vi "Sr530 ChaînePar.vi"(8 "entrée d'erreur (pas d'erreur)":errorcluster, 11 "LockInPar":T1={"BandFilter"=FALSE, "LineFilter1x"=FALSE, "LineFilter2x"=FALSE, "Expand Ch1"=FALSE, "Expand Ch2"=FALSE, "Sensitivity"=1, "Pre Time"=1, "Post Time"=0, "Dynamic Res."=0, "Reference Trigger"=0, "Channels Settings"=0, "Frequency"=0.0} caption="Lock-In Parameters" {"Channels Settings" items=["X, Y", "X Offset, Y Offset", "R, Teta", "R Offset, Teta", "X Noise, Y Noise", "X5 (D/A), X6 (D/A)"]; "Reference Trigger" items=["Positive", "Symmetric", "Negative"]; "Post Time" items=["None", "0.1 s", "1 s"]; "Pre Time" items=["1 ms"=1, "3 ms"=2, "10 ms"=3, "30 ms"=4, "100 ms"=5, "300 ms"=6, "1 s"=7, "3 s"=8, "10 s"=9, "30 s"=10, "100 s"=11]; "Sensitivity" items=["10 nV"=1, "20 nV"=2, "50 nV"=3, "100 nV"=4, "200 nV"=5, "500 nV"=6, "1 µV"=7, "2 µV"=8, "5 µV"=9, "10 µV"=10, "20 µV"=11, "50 µV"=12, "100µV"=13, "200 µV"=14, "500µV"=15, "1 mV"=16, "2 mV"=17, "5 mV"=18, "10 mV"=19, "20 mV"=20, "50 mV"=21, "100 mV"=22]; "Dynamic Res." items=["Low", "Normal", "High"]}) -> (0 "sortie d'erreur":errorcluster, 3 "Chaîne":string)   [LabVIEW 2019]
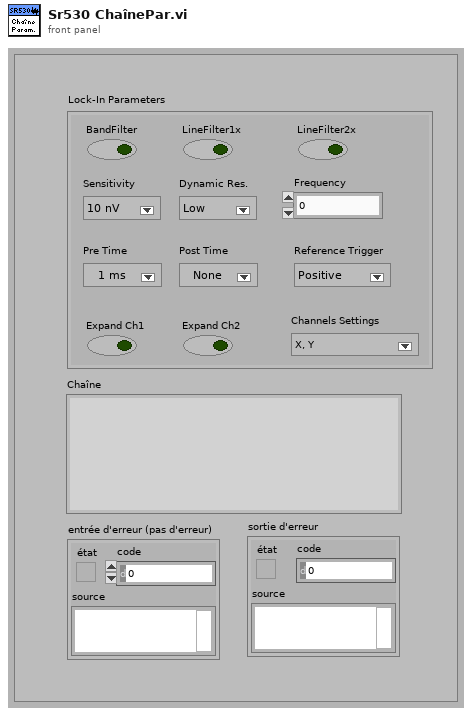
[diagram p1: front panel]
types:
  T1 = cluster{"BandFilter":bool, "LineFilter1x":bool, "LineFilter2x":bool, "Expand Ch1":bool, "Expand Ch2":bool, "Sensitivity":u16, "Pre Time":u16, "Post Time":u16, "Dynamic Res.":u16, "Reference Trigger":u16, "Channels Settings":u16, "Frequency":dbl}
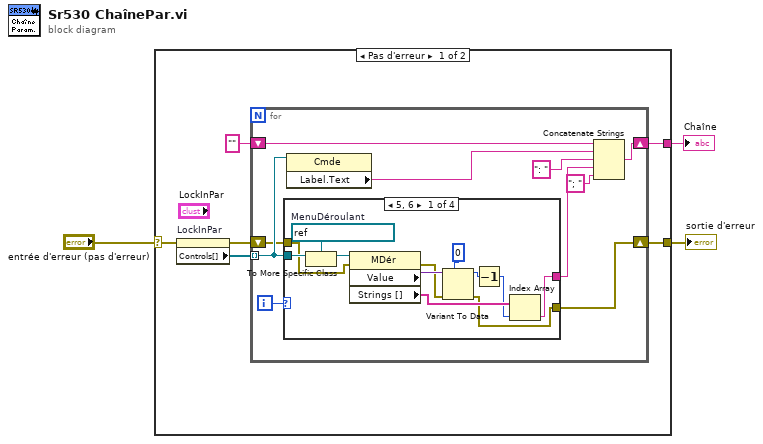
[diagram p0: block diagram]
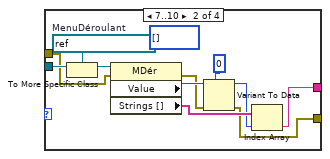
[diagram p2: hidden frame]
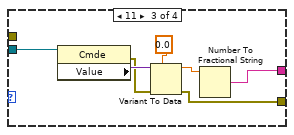
[diagram p3: hidden frame]
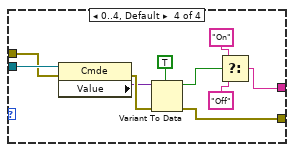
[diagram p4: hidden frame]
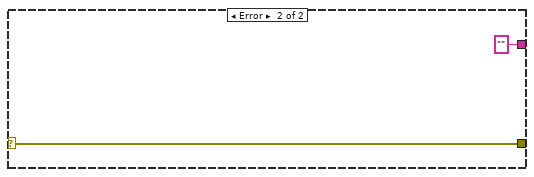
[diagram p5: hidden frame]
diagram:
  n1 = case shown="Pas d'erreur" "entrée d'erreur (pas d'erreur)" {
    selector: "entrée d'erreur (pas d'erreur)" -> [w4 w61]
    tunnel: [w7 ""] -> w3
    tunnel: [w5 w61] -> w2
    frame No Error {
      n2 = property on="LockInPar" class="Clust (strict)"(error in=w4) -> (error out=w6:errorcluster, "Controls[]"=w9:refnum<vi>[])  [unwired: 1 in, 1 out]
      n3 = for {
        tunnel: w9 -> [w18] mode=indexing
        shift-right: [w14] -> w7
        shift-left: "" -> [w13]
        shift-right: [w10] -> w5
        shift-left: w6 -> [w11]
        i -> [w19]
        n4 = case shown="5, 6" w19 {
          tunnel: [w20 w38 w45 w53] -> w15
          tunnel: w18 -> [w27 w37 w44 w52]
          tunnel: w11 -> [w23 w33 _ w51]
          tunnel: [w22 w32 w43 w50] -> w10
          frame 5, 6 {
            w26 = refnum<vi> refnum  # MenuDéroulant
            n5 = To More Specific Class(target class=w26, reference=w27) -> (specific class reference=w25:refnum<vi>)  [unwired: 1 in, 1 out]
            n6 = property class="MDér"(reference=w25, error in=w23) -> (error out=w28:errorcluster, "Value"=w29:variant, "Strings []"=w31:string[])  [unwired: 1 out]
            n7 = Variant To Data(error in=w28, type=0, Variant=w29) -> (data=w24:i32, error out=w22:errorcluster)
            n8 = Decrement(x=w24) -> (x-1=w21:i32)
            n9 = Index Array(array=w31, index=w21) -> (element=w20:string)
          }
          frame 7..10 {
            (unwired) i32[] []
            w36 = refnum<vi> refnum  # MenuDéroulant
            n10 = To More Specific Class(target class=w36, reference=w37) -> (specific class reference=w35:refnum<vi>)  [unwired: 1 in, 1 out]
            n11 = property class="MDér"(reference=w35, error in=w33) -> (error out=w39:errorcluster, "Value"=w40:variant, "Strings []"=w42:string[])  [unwired: 1 out]
            n12 = Variant To Data(error in=w39, type=0, Variant=w40) -> (data=w34:i32, error out=w32:errorcluster)
            n13 = Index Array(array=w42, index=w34) -> (element=w38:string)
          }
          frame 11 {
            n14 = property class="Cmde"(reference=w44) -> (error out=w48:errorcluster, "Value"=w49:variant)  [unwired: 1 in, 1 out]
            n15 = Variant To Data(error in=w48, type=0.0, Variant=w49) -> (data=w46:dbl, error out=w43:errorcluster)
            n16 = Number To Fractional String(number=w46) -> (F-format string=w45:string)  [unwired: 3 in]
          }
          frame 0..4, Default {
            n17 = property class="Cmde"(reference=w52, error in=w51) -> (error out=w59:errorcluster, "Value"=w58:variant)  [unwired: 1 out]
            n18 = Variant To Data(error in=w59, type=TRUE, Variant=w58) -> (data=w56:bool, error out=w50:errorcluster)
            n19 = Select(t="On", s=w56, f="Off") -> (s? t:f=w53:string)
          }
        }
        n20 = property class="Cmde"(reference=w18) -> ("Label.Text"=w17:string)  [unwired: 1 in, 2 out]
        n21 = Concatenate Strings(w13, w17, ": " ("chaîne"), w15, "; " ("chaîne")) -> (w14:string)
      }
    }
    frame Error {
    }
  }
  "Chaîne" <- w3
  "sortie d'erreur" <- w2
